vi "Get Resistance String (SubVI).vi"(8 "Multiplier":u16, 9 "Format String":string, 10 "Resistance Value":i32) -> (2 "Resistance String":string)   [LabVIEW 2011]
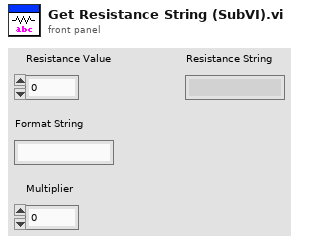
[diagram p1: front panel]
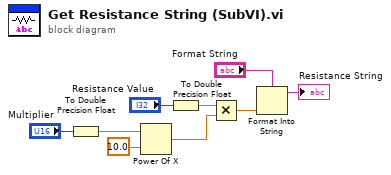
[diagram p0: block diagram]
diagram:
  n1 = To Double Precision Float(number="Multiplier") -> (double precision float=w9:dbl)
  n2 = Power Of X(1:10.0 ("x"), 2:w9) -> (0:w3:dbl)
  n3 = To Double Precision Float(number="Resistance Value") -> (double precision float=w8:dbl)
  n4 = Multiply(x=w8, y=w3) -> (x*y=w5:dbl)
  n5 = Format Into String(format string="Format String", w5) -> (resulting string=→"Resistance String":string)  [unwired: 2 in, 1 out]
